vi "getResults.vi"(0 "reference in":refnum<class "subject.lvclass">, 2 "resultsType":T1, 5 "error in (no error)":errorcluster) -> (14 "reference out":refnum<class "subject.lvclass">, 19 "error out":errorcluster)   [LabVIEW 2015, in "subject.lvclass"]
uses:
  subject.lvclass
  resultsType.ctl
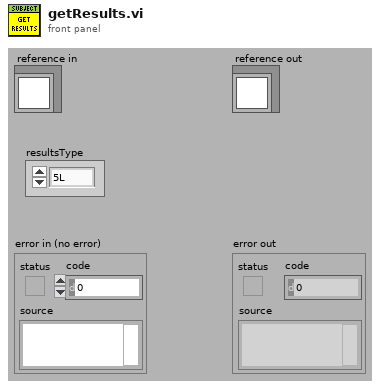
[diagram p1: front panel]
types:
  T1 = typedef "subject.lvclass/resultsType.ctl" = enum16{"5L", "15%", "User Selection"}
  T2 = typedef "subject.lvclass/ObjectAttributesRef.ctl" = refnum<data-value>
  T3 = typedef "subject.lvclass/ObjectAttributes.ctl" = cluster{"MyAttribute":dbl, "data":cluster{"Ve_warm":dbl[], "time_warm":dbl[], "name":string, "phase":dbl[], "VCO2":dbl[], "VO2":dbl[], "PetCO2":dbl[], "RQ":dbl[], "HR":dbl[], "Ve_warm_inter":dbl[], "time_warm_inter":dbl[], "Ve_exer":dbl[], "time_exer":dbl[], "Ve_exer_inter":dbl[], "time_exer_inter":dbl[], "Ve":dbl[], "time":dbl[]}, "results_5l":cluster{"EOV":bool, "osci_amplitude":dbl[], "osci_width":dbl[], "peak_location":dbl[], "threshold":dbl, "width":i32}, "results_15percent":cluster{"EOV":bool, "osci_amplitude":dbl[], "osci_width":dbl[], "peak_location":dbl[], "threshold":dbl, "width":i32}, "supportData":cluster{"peaksAmplitude":dbl[], "iPeaksLocation":dbl[], "valesAmplitude":dbl[], "iValesLocation":dbl[], "threshold":dbl, "meanAmpl_warm":i32, "#_peaks":i32, "width":i32}, "results_user_selection":cluster{"EOV":bool, "osci_amplitude":dbl[], "osci_width":dbl[], "peak_location":dbl[], "threshold":dbl, "width":i32}}
  T4 = cluster{"peaksAmplitude":dbl[], "iPeaksLocation":dbl[], "valesAmplitude":dbl[], "iValesLocation":dbl[], "threshold":dbl, "meanAmpl_warm":i32, "#_peaks":i32, "width":i32}
  T5 = cluster{"EOV":bool, "osci_amplitude":dbl[], "osci_width":dbl[], "peak_location":dbl[], "threshold":dbl, "width":i32}
  T6 = cluster{"Ve_warm":dbl[], "time_warm":dbl[], "name":string, "phase":dbl[], "VCO2":dbl[], "VO2":dbl[], "PetCO2":dbl[], "RQ":dbl[], "HR":dbl[], "Ve_warm_inter":dbl[], "time_warm_inter":dbl[], "Ve_exer":dbl[], "time_exer":dbl[], "Ve_exer_inter":dbl[], "time_exer_inter":dbl[], "Ve":dbl[], "time":dbl[]}
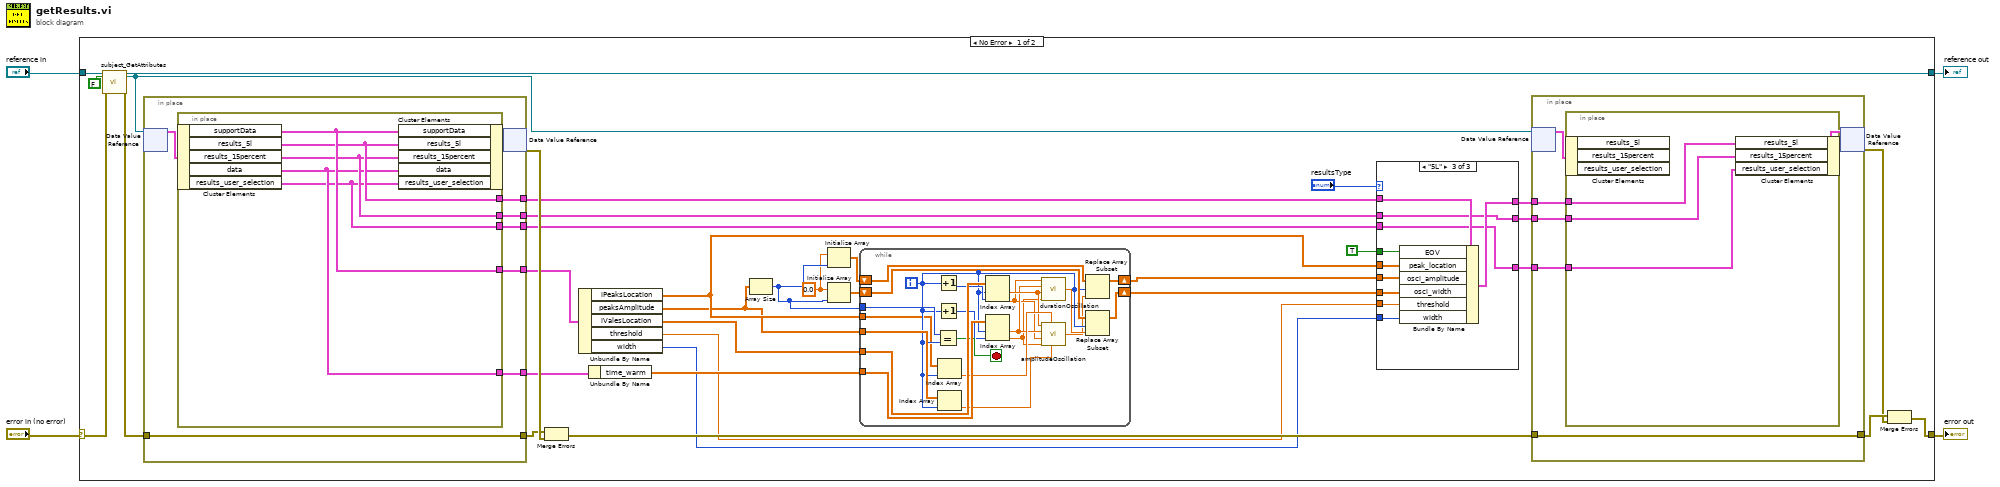
[diagram p0: block diagram]
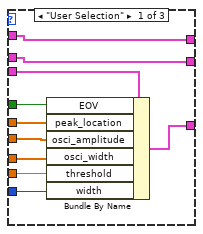
[diagram p2: hidden frame]
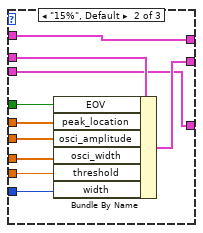
[diagram p3: hidden frame]
diagram:
  n1 = case shown="No Error" "error in (no error)" {
    selector: "error in (no error)" -> [w34 w113]
    tunnel: [w29 w113] -> w3
    tunnel: [w32 w112] -> w1
    tunnel: "reference in" -> [w36 w112]
    frame No Error {
      w18 = 0.0 ("element")
      n2 = call "subject_GetAttributes.vi"("reference in"=w36, "return data? (T)"=FALSE, "error in (no error)"=w34) -> ("reference out"=w32:refnum<class "subject.lvclass">, "attributes ref"=w22:T2, "error out"=w33:errorcluster)  [unwired: 13 in, 1 out]
      n3 = in-place {
        in-place-border: w33 -> [w104]
        in-place-border: [w104] -> w37
        in-place-border: [w103] -> w16
        in-place-border: [w102] -> w27
        in-place-border: [w101] -> w26
        in-place-border: [w100] -> w15
        in-place-border: [w99] -> w8
        n4 = in-place-dvr #1(w22) -> (w105:T3)  [unwired: 1 out]
        n5 = in-place {
          in-place-border: [w111] -> w103
          in-place-border: [w110] -> w102
          in-place-border: [w109] -> w101
          in-place-border: [w108] -> w100
          in-place-border: [w107] -> w99
          n6 = in-place-cluster #2(w105) -> ("supportData"=w111:T4, "results_5l"=w110:T5, "results_15percent"=w109:T5, "data"=w108:T6, "results_user_selection"=w107:T5)
          n7 = in-place-cluster #2("supportData"=w111, "results_5l"=w110, "results_15percent"=w109, "data"=w108, "results_user_selection"=w107) -> (w106:T3)
        }
        n8 = in-place-dvr #1(w106) -> (w38:errorcluster)  [unwired: 1 out]
      }
      n9 = Merge Errors(w37, w38) -> (w13:errorcluster)
      n10 = Unbundle By Name(w16) -> ("iPeaksLocation"=w12:dbl[], "peaksAmplitude"=w7:dbl[], "iValesLocation"=w17:dbl[], "threshold"=w6:dbl, "width"=w5:i32)
      n11 = Unbundle By Name(w15) -> ("time_warm"=w14:dbl[])
      n12 = Array Size(array=w7) -> (size(s)=w21:i32)
      n13 = Initialize Array(w18, w21) -> (w19:dbl[])
      n14 = Initialize Array(w18, w21) -> (w20:dbl[])
      n15 = while {
        tunnel: w7 -> [w59]
        tunnel: w12 -> [w39]
        tunnel: w14 -> [w58]
        tunnel: w17 -> [w57]
        tunnel: w21 -> [w56]
        shift-right: [w49] -> w10
        shift-left: w20 -> [w50]
        shift-right: [w51] -> w11
        shift-left: w19 -> [w52]
        i -> [w48]
        stop <- w55 stop-if-true
        n16 = Equal?(x=w56, y=w48) -> (x = y?=w55:bool)
        n17 = Increment(x=w48) -> (x+1=w53:i32)
        n18 = Increment(x=w48) -> (x+1=w54:i32)
        n19 = Index Array(array=w39, index=w48) -> (element=w46:dbl)
        n20 = Index Array(array=w59, index=w48) -> (element=w45:dbl)
        n21 = Index Array(array=w57, index #1=w48, index #2=w53) -> (element #1=w44:dbl, element #2=w42:dbl)
        n22 = Index Array(array=w58, index #1=w48, index #2=w54) -> (element #1=w43:dbl, element #2=w41:dbl)
        n23 = call "durationOscillation.vi"("valesAmplitude2"=w41, "timeValesLocation1"=w44, "valesAmplitude1"=w43, "timeValesLocation2"=w42) -> ("durationOscilation"=w47:dbl)
        n24 = call "amplitudeOscillation.vi"("y0"=w45, "x0"=w46, "y2"=w41, "x2"=w42, "y1"=w43, "x1"=w44) -> ("amplitudeOscillation"=w40:dbl)
        n25 = Replace Array Subset(array=w52, new element=w40, index=w48) -> (w51:dbl[])
        n26 = Replace Array Subset(array=w50, new element=w47, index=w48) -> (w49:dbl[])
      }
      n27 = case shown="\"5L\"" "resultsType" {
        tunnel: w27 -> [w65 w77 w89]
        tunnel: w26 -> [w66 w79 w87]
        tunnel: [w66 w78 w87] -> w24
        tunnel: [w65 w77 w88] -> w25
        tunnel: TRUE -> [w62 w76 w86]
        tunnel: w12 -> [w67 w75 w85]
        tunnel: w11 -> [w64 w74 w84]
        tunnel: w10 -> [w63 w73 w83]
        tunnel: [w69 w72 w82] -> w9
        tunnel: w8 -> [w68 w72 w82]
        tunnel: w6 -> [w61 w71 w81]
        tunnel: w5 -> [w60 w70 w80]
        frame "User Selection" {
          n28 = Bundle By Name(cluster=w68, "EOV"=w62, "peak_location"=w67, "osci_amplitude"=w64, "osci_width"=w63, "threshold"=w61, "width"=w60) -> (w69:T5)
        }
        frame "15%", Default {
          n29 = Bundle By Name(cluster=w79, "EOV"=w76, "peak_location"=w75, "osci_amplitude"=w74, "osci_width"=w73, "threshold"=w71, "width"=w70) -> (w78:T5)
        }
        frame "5L" {
          n30 = Bundle By Name(cluster=w89, "EOV"=w86, "peak_location"=w85, "osci_amplitude"=w84, "osci_width"=w83, "threshold"=w81, "width"=w80) -> (w88:T5)
        }
      }
      n31 = in-place {
        in-place-border: w13 -> [w93]
        in-place-border: [w93] -> w31
        in-place-border: w25 -> [w92]
        in-place-border: w24 -> [w91]
        in-place-border: w9 -> [w90]
        n32 = in-place-dvr #3(w22) -> (w94:T3)  [unwired: 1 out]
        n33 = in-place {
          in-place-border: w92 -> [w98]
          in-place-border: w91 -> [w97]
          in-place-border: w90 -> [w96]
          n34 = in-place-cluster #4(w94) -> ()  [unwired: 3 out]
          n35 = in-place-cluster #4("results_5l"=w98, "results_15percent"=w97, "results_user_selection"=w96) -> (w95:T3)
        }
        n36 = in-place-dvr #3(w95) -> (w30:errorcluster)  [unwired: 1 out]
      }
      n37 = Merge Errors(w31, w30) -> (w29:errorcluster)
    }
    frame Error {
    }
  }
  "error out" <- w3
  "reference out" <- w1
